vi "MISC Search 2D Array.vi"(0 "Array":dbl[][](array[numeric]) format="%.2f", 5 "Element":dbl format="%.2f") -> (4 "Row":i32, 6 "Column":i32)   [LabVIEW 2011]
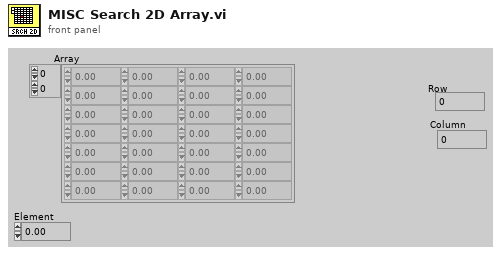
[diagram p1: front panel]
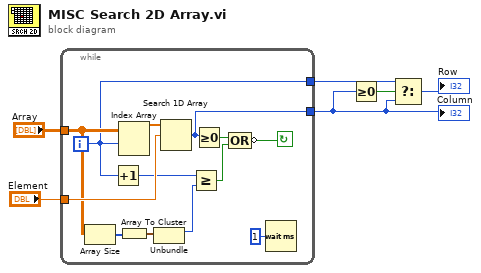
[diagram p0: block diagram]
diagram:
  n1 = while {
    tunnel: [w13] -> w4
    tunnel: [w17] -> w1
    tunnel: "Element" -> [w18]
    tunnel: "Array" -> [w16]
    i -> [w13]
    stop <- w7 continue-if-true
    n2 = Array Size(array=w16) -> (size(s)=w14:i32[])
    n3 = Increment(x=w13) -> (x+1=w15:i32)
    n4 = Index Array(array=w16, index (row)=w13) -> (element=w19:dbl[])  [unwired: 1 in]
    n5 = Array To Cluster(array=w14) -> (cluster=w10:cluster{"[0]":i32, "[1]":i32})
    n6 = Unbundle(w10) -> ("[0]"=w9:i32)  [unwired: 1 out]
    n7 = Search 1D Array(1D array=w19, element=w18) -> (index of element=w17:i32)  [unwired: 1 in]
    n8 = Greater Or Equal?(x=w15, y=w9) -> (x >= y?=w11:bool)
    n9 = Greater Or Equal To 0?(x=w17) -> (x >= 0?=w12:bool)
    n10 = Compound Arithmetic op=OR(w12, w11) -> (invert w7:bool)
    n11 = Wait (ms)(milliseconds to wait=u32 1) -> ()  [unwired: 1 out]
  }
  "Column" <- w1
  n12 = Greater Or Equal To 0?(x=w1) -> (x >= 0?=w2:bool)
  n13 = Select(t=w4, s=w2, f=w1) -> (s? t:f=→"Row":i32)
